vi "Supported Smart Syntax Representation.vi"(0 "Booelan Operations in":refnum<class "Boolean Functions.lvclass">, 11 "error in (no error)":errorcluster) -> (4 "Booelan Operations out":refnum<class "Boolean Functions.lvclass">, 6 "Smart Syntax Representation List":string[](array[string]), 15 "error out":errorcluster)   [LabVIEW 2019, in "Boolean Functions.lvclass"]
uses:
  Boolean Functions.lvclass
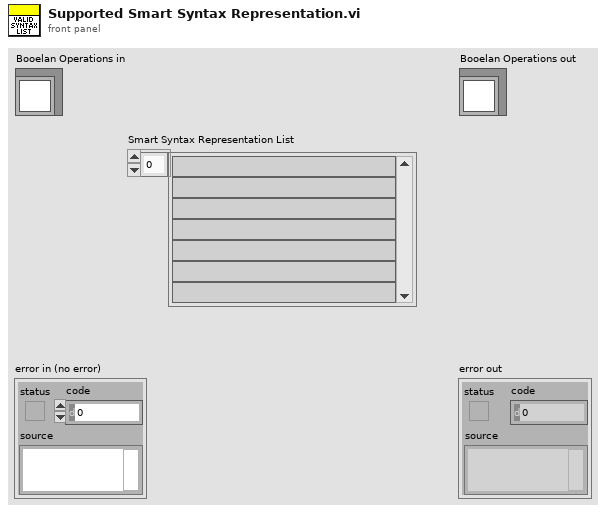
[diagram p1: front panel]
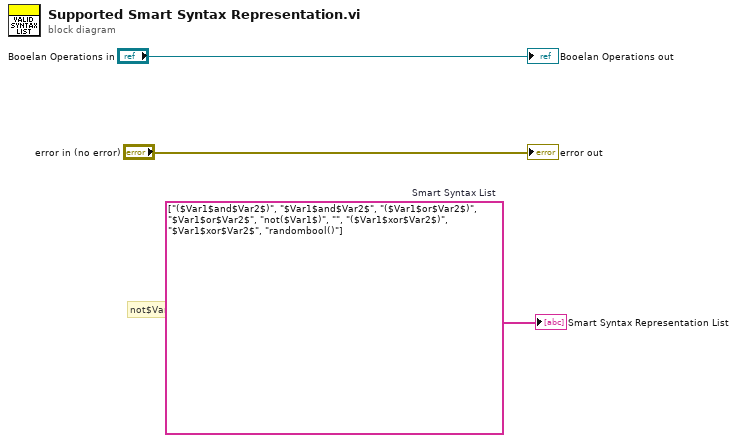
[diagram p0: block diagram]
diagram:
  w1 = string[] ["($Var1$and$Var2$)", "$Var1$and$Var2$", "($Var1$or$Var2$)", "$Var1$or$Var2$", "not($Var1$)", "", "($Var1$xor$Var2$)", "$Var1$xor$Var2$", "randombool()"]  # Smart Syntax List
  # "not$Var1$"
  "error out" <- "error in (no error)"
  "Booelan Operations out" <- "Booelan Operations in"
  "Smart Syntax Representation List" <- w1
